vi "Left SPI Sample and Parse (SubVI).vi"(5 "SPI Ref In":T1={"myRIO Reference"={"myRIO Model"=enum."Unknown", "myRIO Hardware Reference"={"Generic FPGA Reference"=refnum, "Allow multiple opens"=FALSE}}, "SPI Channels Enum"=enum."Not Connected", "SPI Configuration"={"Frequency [Hz]"=0.0, "Clock Phase"=enum."Leading", "Clock Polarity"=enum."Low", "Data Direction"=enum."Most significant bit first", "Frame Length"=8}} {"SPI Configuration"."Frame Length" min=1 max=16}) -> (0 "Two Beacons Seen?":bool, 1 "o2 Checksum OK?":bool, 2 "o1 Checksum OK?":bool)   [LabVIEW 2015]
uses:
  <vilib>/myRIO/Instrument Drivers/Onboard IO/SPI/typedefs/SPI Reference.ctl
  <vilib>/myRIO/Common/Instrument Driver Framework/Utilities/typedefs/myRIO Generic Hardware Reference.ctl
  <vilib>/myRIO/Common/Instrument Driver Framework/Utilities/typedefs/Hardware Version Enum.ctl
  <vilib>/myRIO/Common/Instrument Driver Framework/Utilities/typedefs/myRIO v1.0 Reference.ctl
  <vilib>/myRIO/Common/Instrument Driver Framework/Utilities/typedefs/Generic FPGA Reference.ctl
  <vilib>/myRIO/Common/Instrument Driver Framework/myRIO v1.0/SPI/typedefs/SPI Channels Enum.ctl
  <vilib>/myRIO/Instrument Drivers/Onboard IO/SPI/typedefs/SPI Configuration.ctl
  <vilib>/myRIO/Common/Instrument Driver Framework/myRIO v1.0/SPI/typedefs/SPI Clock Phase.ctl
  <vilib>/myRIO/Common/Instrument Driver Framework/myRIO v1.0/SPI/typedefs/SPI Clock Polarity.ctl
  <vilib>/myRIO/Common/Instrument Driver Framework/myRIO v1.0/SPI/typedefs/SPI Data Direction.ctl
  <vilib>/myRIO/Common/Instrument Driver Framework/myRIO v1.0/SPI/typedefs/SPI Frame Length.ctl
  <vilib>/myRIO/Instrument Drivers/Onboard IO/SPI/vis/Write Read.vi
  <vilib>/Utility/error.llb/Error Cluster From Error Code.vi
  <vilib>/myRIO/Common/Instrument Driver Framework/myRIO v1.0/SPI/vis/myRIO v1.0 Write Read SPI.vi
  Left Variables.vi
  <vilib>/myRIO/Instrument Drivers/Onboard IO/SPI/SPI.lvlib
panel:
  out "String":string
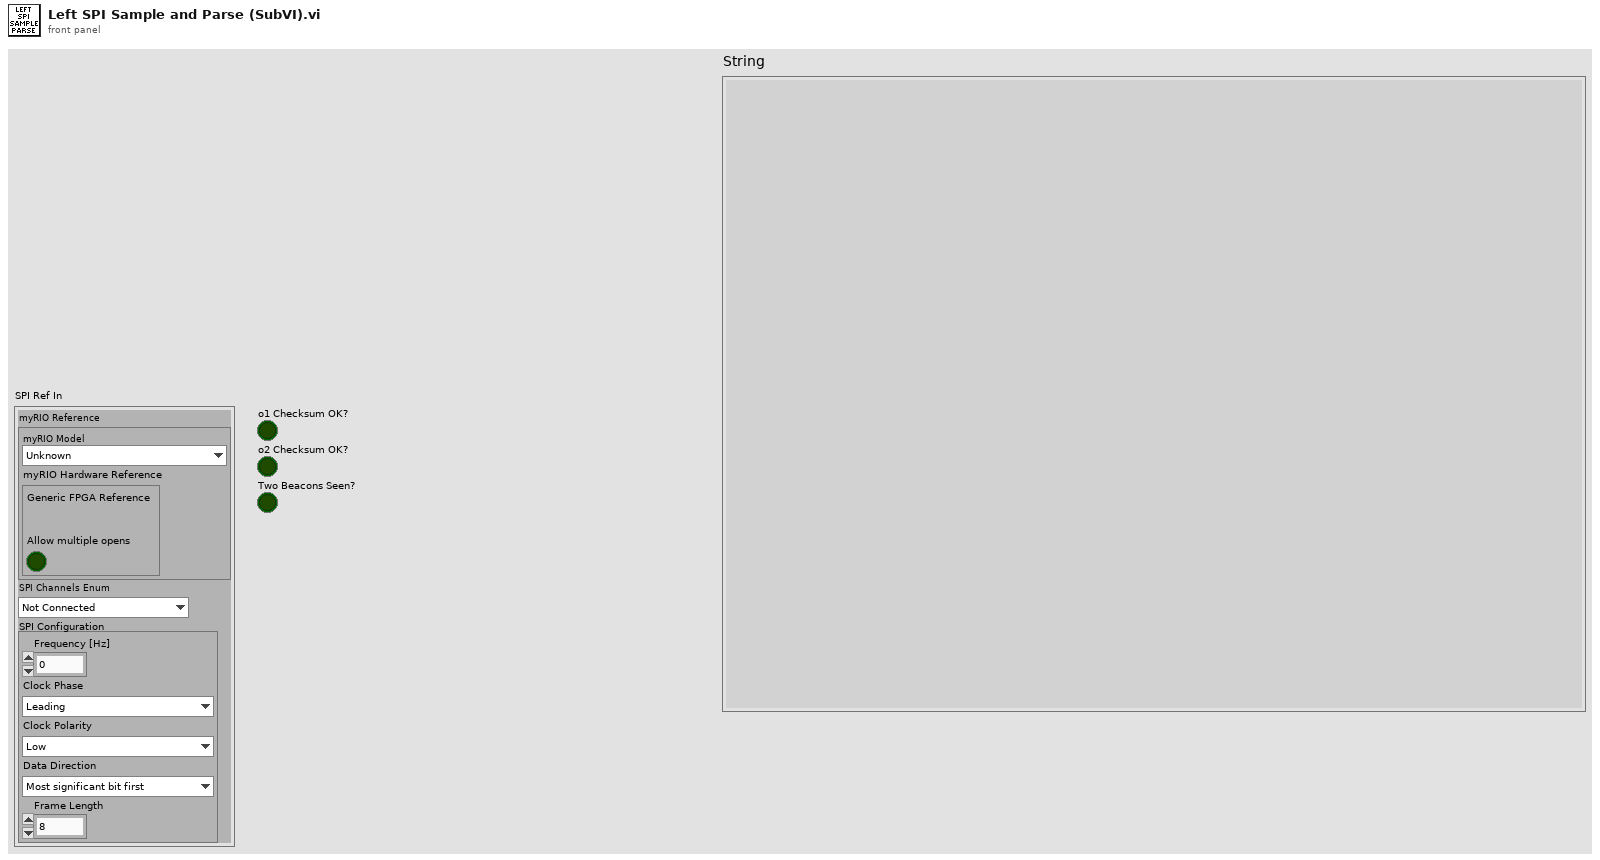
[diagram p1: front panel]
types:
  T1 = typedef "SPI.lvlib/SPI Reference.ctl" = cluster{"myRIO Reference":T2, "SPI Channels Enum":T6, "SPI Configuration":T7}
  T2 = typedef "myRIO Generic Hardware Reference.ctl" = cluster{"myRIO Model":T3, "myRIO Hardware Reference":T4}
  T3 = typedef "Hardware Version Enum.ctl" = enum16{"Unknown", "myRIO-1900", "myRIO-1950", "roboRIO"}
  T4 = typedef "myRIO v1.0 Reference.ctl" = cluster{"Generic FPGA Reference":T5, "Allow multiple opens":bool}
  T5 = typedef "Generic FPGA Reference.ctl" = refnum<k20>
  T6 = typedef "SPI Channels Enum.ctl" = enum16{"Not Connected", "A/SPI", "B/SPI", "SPI/SPI"}
  T7 = typedef "SPI.lvlib/SPI Configuration.ctl" = cluster{"Frequency [Hz]":dbl, "Clock Phase":T8, "Clock Polarity":T9, "Data Direction":T10, "Frame Length":T11}
  T8 = typedef "SPI Clock Phase.ctl" = enum8{"Leading", "Trailing"}
  T9 = typedef "SPI Clock Polarity.ctl" = enum8{"Low", "High"}
  T10 = typedef "SPI Data Direction.ctl" = enum8{"Most significant bit first", "Least significant bit first"}
  T11 = typedef "SPI Frame Length.ctl" = u8
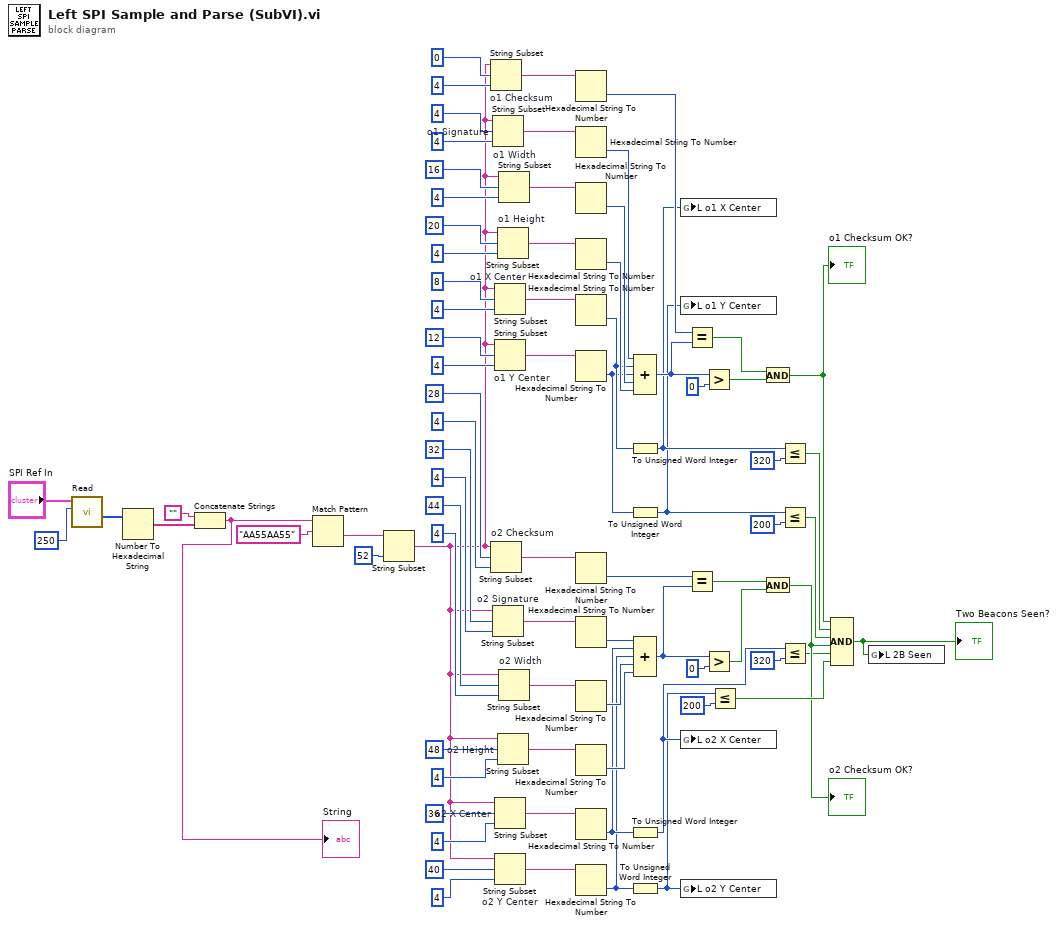
[diagram p0: block diagram]
diagram:
  n1 = call <vilib>:"Read.vi"("Frame Count"=u32 250, "SPI Ref In"="SPI Ref In") -> ("Frames Read"=w3:u16[])  [unwired: 6 in, 2 out]
  n2 = Number To Hexadecimal String(2:w3) -> (0:w2:string[])  [unwired: 1 in]
  n3 = Concatenate Strings("", w2) -> (w1:string)
  "String" <- w1
  n4 = Match Pattern(string=w1, regular expression="AA55AA55") -> (after substring=w20:string)  [unwired: 1 in, 3 out]
  n5 = String Subset(string=w20, length (rest)=52 ("length (rest)")) -> (substring=w18:string)  [unwired: 1 in]
  n6 = String Subset "o1 Checksum"(string=w18, offset (0)=0, length (rest)=4 ("length (rest)")) -> (substring=w59:string)
  n7 = String Subset "o2 Checksum"(string=w18, offset (0)=28, length (rest)=4 ("length (rest)")) -> (substring=w79:string)
  n8 = String Subset "o1 Signature"(string=w18, offset (0)=4, length (rest)=4 ("length (rest)")) -> (substring=w57:string)
  n9 = String Subset "o2 Signature"(string=w18, offset (0)=32, length (rest)=4 ("length (rest)")) -> (substring=w78:string)
  n10 = String Subset "o1 X Center"(string=w18, offset (0)=8, length (rest)=4 ("length (rest)")) -> (substring=w56:string)
  n11 = String Subset "o1 Y Center"(string=w18, offset (0)=12, length (rest)=4 ("length (rest)")) -> (substring=w55:string)
  n12 = String Subset "o2 X Center"(string=w18, offset (0)=36, length (rest)=4 ("length (rest)")) -> (substring=w77:string)
  n13 = String Subset "o2 Y Center"(string=w18, offset (0)=40, length (rest)=4 ("length (rest)")) -> (substring=w76:string)
  n14 = String Subset "o1 Height"(string=w18, offset (0)=20, length (rest)=4 ("length (rest)")) -> (substring=w53:string)
  n15 = String Subset "o2 Height"(string=w18, offset (0)=48, length (rest)=4 ("length (rest)")) -> (substring=w74:string)
  n16 = String Subset "o1 Width"(string=w18, offset (0)=16, length (rest)=4 ("length (rest)")) -> (substring=w54:string)
  n17 = String Subset "o2 Width"(string=w18, offset (0)=44, length (rest)=4 ("length (rest)")) -> (substring=w75:string)
  n18 = Hexadecimal String To Number(string=w59) -> (number=w36:u32)  [unwired: 2 in, 1 out]
  n19 = Hexadecimal String To Number(string=w57) -> (number=w58:u32)  [unwired: 2 in, 1 out]
  n20 = Hexadecimal String To Number(string=w54) -> (number=w60:u32)  [unwired: 2 in, 1 out]
  n21 = Hexadecimal String To Number(string=w53) -> (number=w61:u32)  [unwired: 2 in, 1 out]
  n22 = Hexadecimal String To Number(string=w56) -> (number=w35:u32)  [unwired: 2 in, 1 out]
  n23 = Hexadecimal String To Number(string=w55) -> (number=w34:u32)  [unwired: 2 in, 1 out]
  n24 = Hexadecimal String To Number(string=w79) -> (number=w39:u32)  [unwired: 2 in, 1 out]
  n25 = Hexadecimal String To Number(string=w78) -> (number=w40:u32)  [unwired: 2 in, 1 out]
  n26 = Hexadecimal String To Number(string=w75) -> (number=w80:u32)  [unwired: 2 in, 1 out]
  n27 = Hexadecimal String To Number(string=w74) -> (number=w81:u32)  [unwired: 2 in, 1 out]
  n28 = Hexadecimal String To Number(string=w77) -> (number=w38:u32)  [unwired: 2 in, 1 out]
  n29 = Hexadecimal String To Number(string=w76) -> (number=w37:u32)  [unwired: 2 in, 1 out]
  n30 = To Unsigned Word Integer(number=w35) -> (unsigned 16bit integer=w10:u16)
  n31 = To Unsigned Word Integer(number=w34) -> (unsigned 16bit integer=w9:u16)
  n32 = To Unsigned Word Integer(number=w38) -> (unsigned 16bit integer=w8:u16)
  n33 = To Unsigned Word Integer(number=w37) -> (unsigned 16bit integer=w7:u16)
  n34 = Compound Arithmetic op=ADD(w58, w35, w34, w60, w61) -> (w24:u32)
  n35 = Compound Arithmetic op=ADD(w40, w38, w37, w80, w81) -> (w30:u32)
  n36 = global write "Left Variables.vi" "L o1 X Center"(w10) -> ()
  n37 = global write "Left Variables.vi" "L o1 Y Center"(w9) -> ()
  n38 = global write "Left Variables.vi" "L o2 X Center"(w8) -> ()
  n39 = global write "Left Variables.vi" "L o2 Y Center"(w7) -> ()
  n40 = Equal?(x=w36, y=w24) -> (x = y?=w23:bool)
  n41 = Equal?(x=w39, y=w30) -> (x = y?=w27:bool)
  n42 = Greater?(x=w24, y=u32 0) -> (0:w25:bool)
  n43 = Greater?(x=w30, y=u32 0) -> (0:w28:bool)
  n44 = Less Or Equal?(x=w7, y=u16 200) -> (x <= y?=w31:bool)
  n45 = And(x=w23, y=w25) -> (x .and. y?=w22:bool)
  "o1 Checksum OK?" <- w22
  n46 = And(x=w27, y=w28) -> (x .and. y?=w14:bool)
  "o2 Checksum OK?" <- w14
  n47 = Less Or Equal?(x=w10, y=u16 320) -> (x <= y?=w12:bool)
  n48 = Less Or Equal?(x=w9, y=u16 200) -> (x <= y?=w11:bool)
  n49 = Less Or Equal?(x=w8, y=u16 320) -> (x <= y?=w13:bool)
  n50 = Compound Arithmetic op=AND(w22, w12, w11, w14, w13, w31) -> (w6:bool)
  "Two Beacons Seen?" <- w6
  n51 = global write "Left Variables.vi" "L 2B Seen"(w6) -> ()
